vi "Configure Temperature1.vi"(6 "Nominal Resistance (100 ohm)":dbl=100.0, 8 "error in (no error)":errorcluster, 9 "Probe Type (0: RTD 4-wire)":i32(ring) items=["RTD 4-wire", "RTD 2-wire", "Thermistor 4-wire", "Thermistor 2-wire"], 10 "Temperature Integration Time (10: 10)":dbl(ring)=10.0 items=["0.02"=0.02, "0.2"=0.2, "1"=1.0, "10"=10.0, "100"=100.0], 11 "VISA resource name":refnum<visa-resource-name>) -> (0 "error out":errorcluster, 3 "VISA resource name out":refnum<visa-resource-name>)   [LabVIEW 2015, in "Agilent 3446X Series1.lvlib"]
doc: "Configures the temperature measurement settings."
uses:
  Agilent 3446X Series1.lvlib
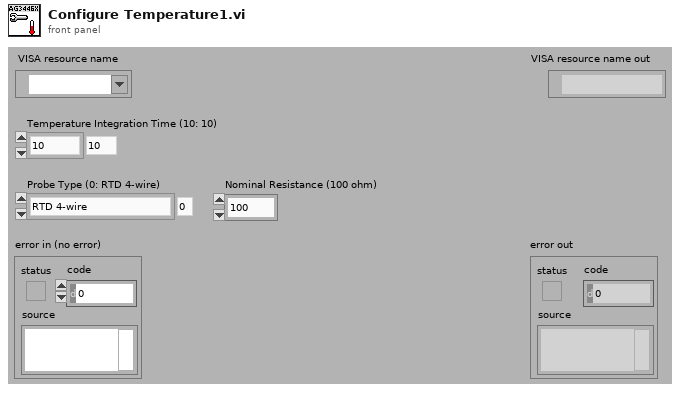
[diagram p1: front panel]
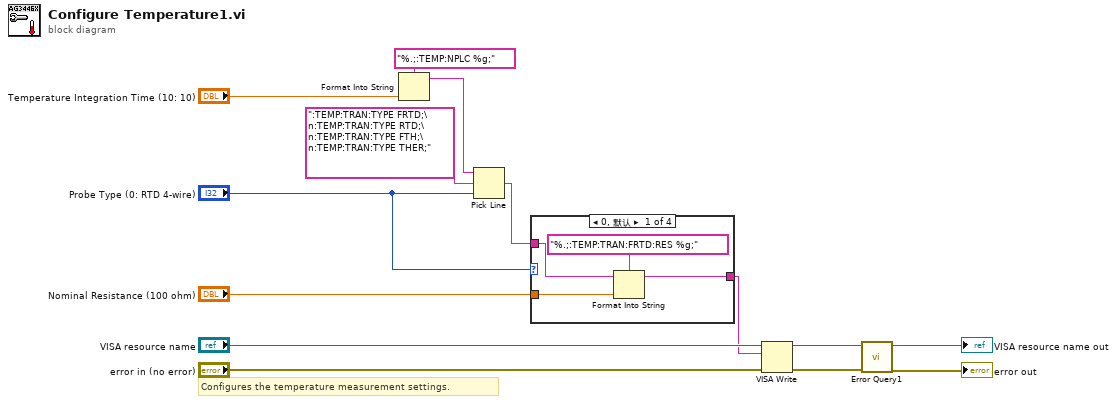
[diagram p0: block diagram]
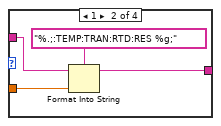
[diagram p2: hidden frame]
diagram:
  # "Configures the temperature measurement settings."
  n1 = Format Into String(format string="%.;:TEMP:NPLC %g;", "Temperature Integration Time (10: 10)") -> (resulting string=w11:string)  [unwired: 2 in, 1 out]
  n2 = Pick Line(string ("")=w11, multi-line string=":TEMP:TRAN:TYPE FRTD;\n:TEMP:TRAN:TYPE RTD;\n:TEMP:TRAN:TYPE FTH;\n:TEMP:TRAN:TYPE THER;", line index="Probe Type (0: RTD 4-wire)") -> (output string=w3:string)
  n3 = case shown="0, 默认" "Probe Type (0: RTD 4-wire)" {
    tunnel: w3 -> [w17 w21 w23 w24]
    tunnel: "Nominal Resistance (100 ohm)" -> [w16 w20 _ _]
    tunnel: [w15 w19 w23 w24] -> w1
    frame 0, Default {
      n4 = Format Into String(format string="%.;:TEMP:TRAN:FRTD:RES %g;", initial string=w17, w16) -> (resulting string=w15:string)  [unwired: 1 in, 1 out]
    }
    frame 1 {
      n5 = Format Into String(format string="%.;:TEMP:TRAN:RTD:RES %g;", initial string=w21, w20) -> (resulting string=w19:string)  [unwired: 1 in, 1 out]
    }
    frame 2 {
    }
    frame 3 {
    }
  }
  n6 = VISA Write(VISA resource name="VISA resource name", write buffer=w1, error in (no error)="error in (no error)") -> (VISA resource name out=w8:refnum<visa-resource-name>, error out=w7:errorcluster)  [unwired: 1 out]
  n7 = call "Error Query1.vi"("error in (no error)"=w7, "VISA resource name"=w8) -> ("error out"=→"error out":errorcluster, "VISA resource name out"=→"VISA resource name out":refnum<visa-resource-name>)  [unwired: 8 out]
